vi "Power Measurement Standard Deviation Error Codes.vi"(8 "error in (no error)":errorcluster, 10 "Instance (1)":i32=1, 11 "VISA resource name":refnum<visa-resource-name>) -> (0 "error out":errorcluster, 1 "Error Codes":i32[](array[numeric]), 2 "Reliability":i32, 3 "VISA resource name out":refnum<visa-resource-name>)   [LabVIEW 2015, in "Rohde&Schwarz CMXP GPRF.lvlib"]
doc: "Returns a single-value error code for each result.\n\nAttribute:\nRSCMXPGPRF_ATTR_POWER_MEASUREMENT_STANDARD_DEVIATION\n\nRemote-control command:\nCALCulate:GPRF:MEAS<i>:POWer:SDEViation?"
uses:
  <instrlib>/Rohde&Schwarz CMXP GPRF/Rohde&Schwarz CMXP GPRF.lvlib
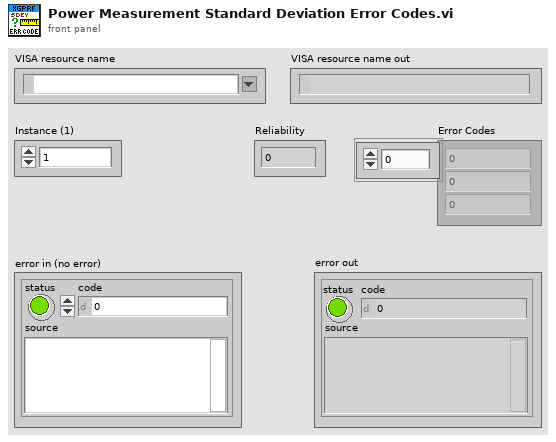
[diagram p1: front panel]
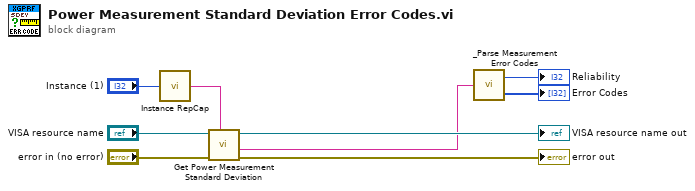
[diagram p0: block diagram]
diagram:
  n1 = call <instrlib>:"Instance RepCap.vi"("instance  in"="Instance (1)") -> ("instance out"=w4:string)
  n2 = call "Get Power Measurement Standard Deviation"("Repeated Capabilities"=w4, "error in (no error)"="error in (no error)", "instrument handle"="VISA resource name") -> ("error out"=→"error out":errorcluster, "Power Measurement Standard Deviation"=w1:string, "instrument handle out"=→"VISA resource name out":refnum<visa-resource-name>)  [unwired: 6 in]
  n3 = call <instrlib>:"_Parse Measurement Error Codes.vi"("String In"=w1) -> ("Reliability"=→"Reliability":i32, "Results"=→"Error Codes":i32[])
